vi "To Float.vi"(10 "Status Message":u8[](array[numeric])) -> (2 "Float":dbl)   [LabVIEW 2018, in "Kronos.lvlib" / "Kronos.lvclass"]
uses:
  Kronos.lvclass
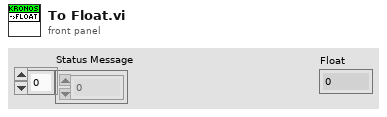
[diagram p1: front panel]
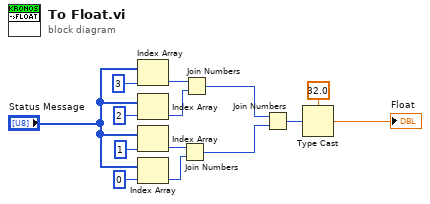
[diagram p0: block diagram]
diagram:
  n1 = Index Array(array="Status Message", index=3) -> (element=w8:u8)
  n2 = Index Array(array="Status Message", index=2) -> (element=w7:u8)
  n3 = Index Array(array="Status Message", index=1) -> (element=w6:u8)
  n4 = Index Array(array="Status Message", index=0) -> (element=w5:u8)
  n5 = Join Numbers(hi=w6, lo=w5) -> ((hi.lo)=w3:u16)
  n6 = Join Numbers(hi=w8, lo=w7) -> ((hi.lo)=w4:u16)
  n7 = Join Numbers(hi=w4, lo=w3) -> ((hi.lo)=w13:u32)
  n8 = Type Cast(type=sgl 32.0, x=w13) -> (*(type *) &x=→"Float":sgl)
